vi "Main Low Level.vi"() -> ()   [LabVIEW 2015]
uses:
  <vilib>/userdefined/High Color/IMAQdx.ctl
  <vilib>/myRIO/Instrument Drivers/Onboard IO/UART/typedef/VISA Configuration.ctl
  <vilib>/Instr/_visa.llb/VISA Configure Serial Port (Instr).vi
  <vilib>/myRIO/Instrument Drivers/Onboard IO/UART/UART.lvlib
  <vilib>/vision/driver/NI_Vision_Acquisition_Software.lvlib
panel:
  out "NEW A":i32
  out "STOP STATE":dbl
  out "FRONT STATE":dbl
  out "LEFT STATE":dbl
  out "RIGHT STATE":dbl
  out "Buffer Number Out":u32
  in  "Session In":T1
  out "break stat":u16
  out "right stat":u16
  out "down stat":u16
  out "left stat":u16
  out "up stat":u16
  in  "stop":bool
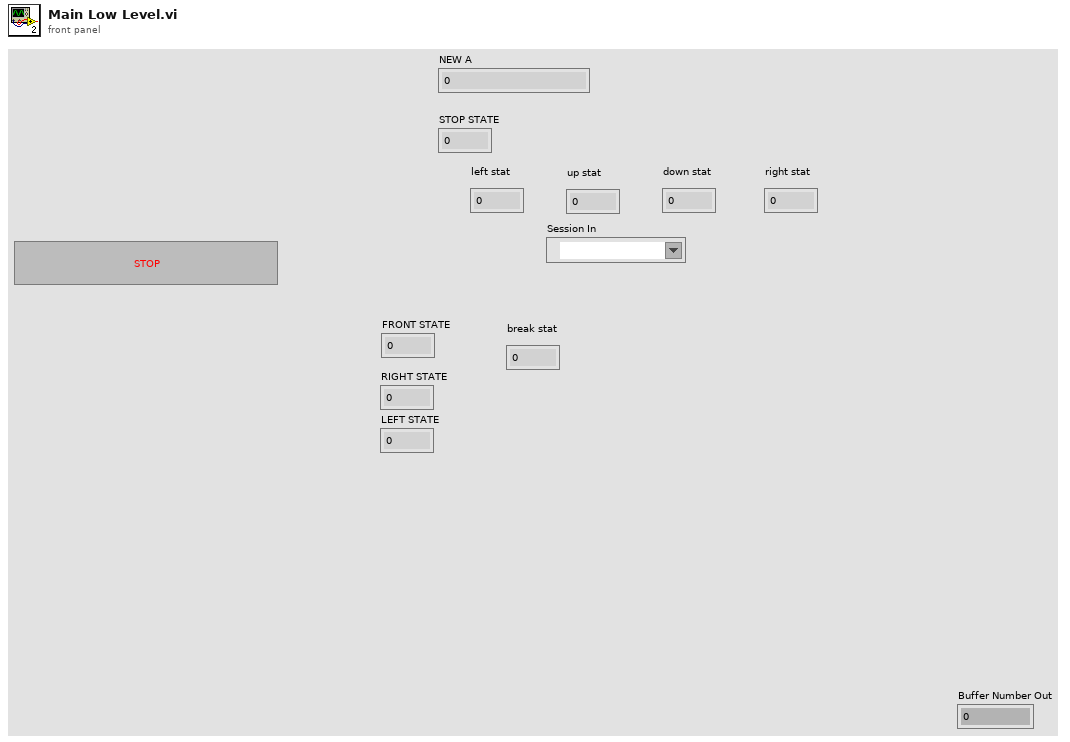
[diagram p1: front panel]
types:
  T1 = typedef "IMAQdx.ctl" = refnum<k21>
  T2 = typedef "Image Type" = u32
  T3 = typedef "UART.lvlib/VISA Configuration.ctl" = cluster{"baud rate (9600)":u32, "data bits (8)":u16, "parity (0:none)":enum16{"None", "Odd", "Even", "Mark", "Space"}, "stop bits (10: 1 bit)":u16, "flow control (0:none)":u16, "termination char\n(0xA = '\\n' = LF) ":u8, "Enable Termination\nChar (T)":bool, "timeout (10sec)":u32}
  T4 = typedef "IMAQ Image.ctl" = refnum<image>
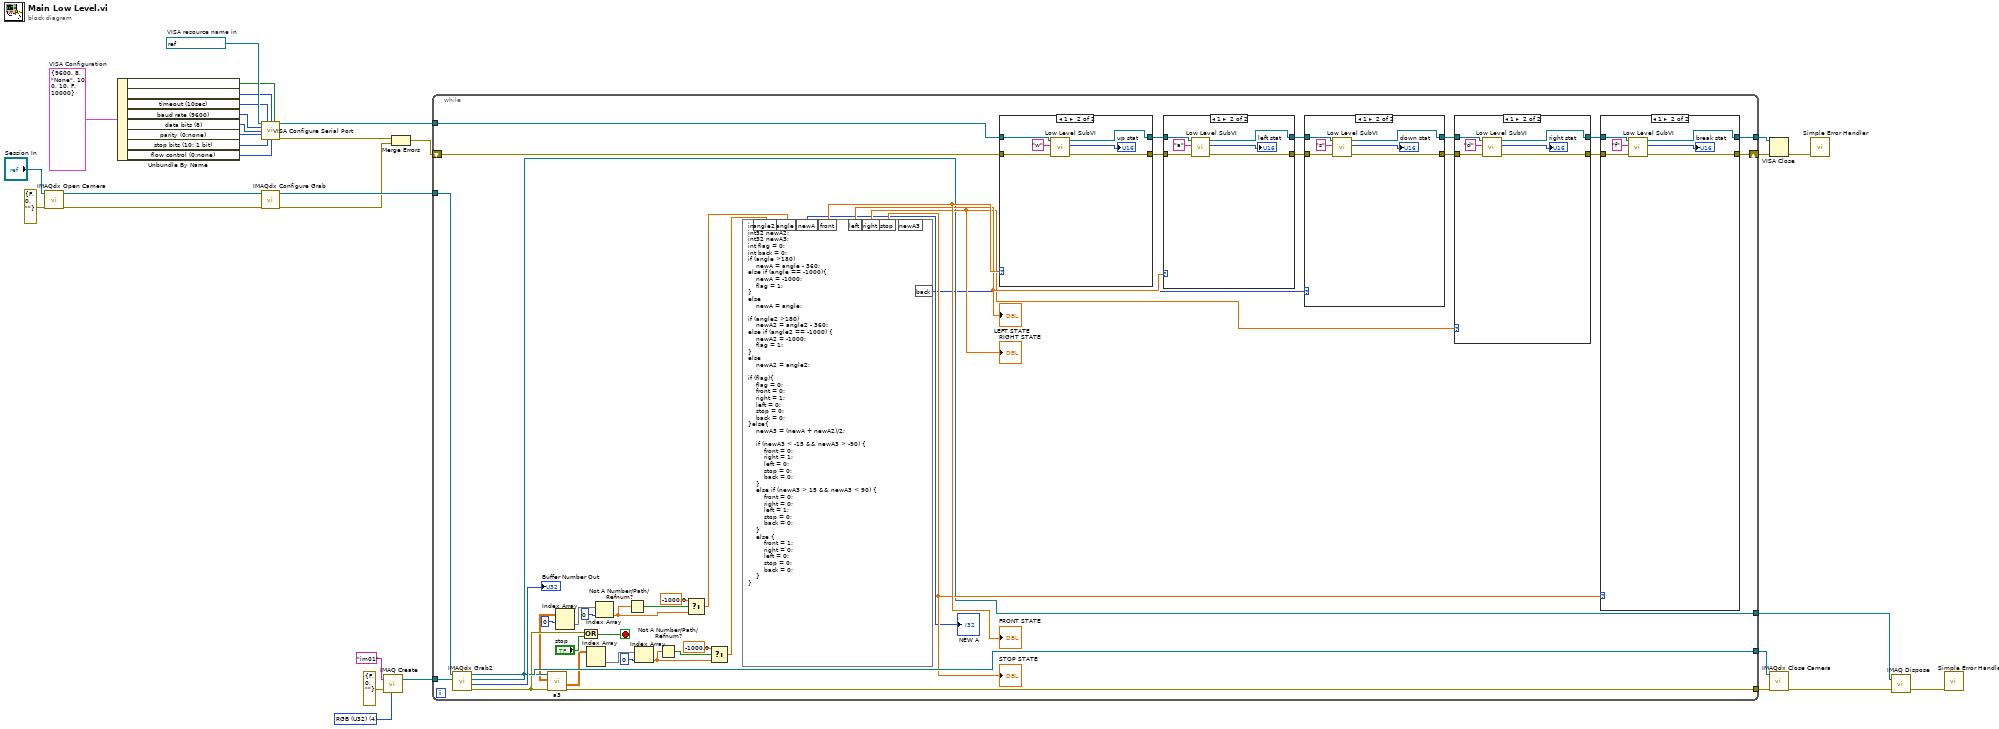
[diagram p0: block diagram]
diagram:
  w13 = T2 4 items=["Grayscale (U8)", "Grayscale (I16)", "Grayscale (SGL)", "Complex (CSG)", "RGB (U32)", "HSL (U32)", "RGB (U64)", "Grayscale (U16)"] ("Image Type")
  w30 = T3 {"baud rate (9600)"=9600, "data bits (8)"=8, "parity (0:none)"=enum."None", "stop bits (10: 1 bit)"=10, "flow control (0:none)"=0, "termination char\n(0xA = '\\n' = LF) "=10, "Enable Termination\nChar (T)"=FALSE, "timeout (10sec)"=10000}  # VISA Configuration
  w31 = refnum<visa-resource-name> "ASRL1::INSTR"  # VISA resource name in
  n1 = call <vilib>:"IMAQdx Open Camera.vi"("error in"=errorcluster {"status"=FALSE, "code"=0, "source"=""}, "Session In"="Session In") -> ("error out"=w16:errorcluster, "Session Out"=w17:T1)  [unwired: 8 in]
  n2 = Unbundle By Name(w30) -> ("Enable Termination\nChar (T)"=w29:bool, "termination char\n(0xA = '\\n' = LF)"=w28:u8, "timeout (10sec)"=w27:u32, "baud rate (9600)"=w22:u32, "data bits (8)"=w23:u16, "parity (0:none)"=w24:enum16{"None", "Odd", "Even", "Mark", "Space"}, "stop bits (10: 1 bit)"=w25:u16, "flow control (0:none)"=w26:u16)
  n3 = call-poly "VISA Configure Serial Port"("VISA resource name"=w31, "timeout (10sec)"=w27, "termination char\n(0xA = '\\n' = LF)"=w28, "Enable Termination\nChar (T)"=w29, "baud rate (9600)"=w22, "data bits (8)"=w23, "parity (0:none)"=w24, "stop bits (10: 1 bit)"=w25, "flow control (0:none)"=w26) -> ("VISA resource name out"=w21:refnum<visa-resource-name>, "error out"=w6:errorcluster)  [unwired: 5 in]
  n4 = call <vilib>:"IMAQdx Configure Grab.vi"("error in"=w16, "Session In"=w17) -> ("error out"=w7:errorcluster, "Session Out"=w8:T1)  [unwired: 8 in]
  n5 = call "IMAQ Create"("Image Name"="im01", "Image Type"=w13, "error in (no error)"=errorcluster {"status"=FALSE, "code"=0, "source"=""}) -> ("New Image"=w4:T4)  [unwired: 2 in, 1 out]
  n6 = Merge Errors(w6, w7) -> (w5:errorcluster)
  n7 = while {
    tunnel: w21 -> [w73]
    shift-right: [w57] -> w20
    shift-left: w5 -> [w72]
    tunnel: [w63] -> w19
    tunnel: w8 -> [w61]
    tunnel: w4 -> [w60]
    tunnel: [w44] -> w3
    tunnel: [w56] -> w2
    tunnel: [w43] -> w1
    stop <- w58 stop-if-true
    n8 = call <vilib>:"IMAQdx Grab2.vi"("Image In"=w60, "Session In"=w61) -> ("error out"=w45:errorcluster, "Buffer Number Out"=→"Buffer Number Out":u32, "Image Out"=w44:T4, "Session Out"=w56:T1)  [unwired: 6 in]
    n9 = call "a3.vi"("error in"=w45, "Image In"=w44) -> ("error out"=w43:errorcluster, "Calibrated Results (Caliper 2)"=w42:sgl[][], "Calibrated Results (Caliper 1)"=w41:sgl[][])  [unwired: 3 out]
    n10 = Index Array(array=w41, index (row)=0) -> (element=w51:sgl[])  [unwired: 1 in]
    n11 = Or(x=w45, y="stop") -> (x .or. y?=w58:bool)
    n12 = Index Array(array=w42) -> (element=w48:sgl[])  [unwired: 2 in]
    n13 = Index Array(array=w51, index=0) -> (element=w35:sgl)
    n14 = Not A Number/Path/Refnum?(number/path/refnum=w35) -> (NaN/Path/Refnum?=w36:bool)
    n15 = Index Array(array=w48, index=0) -> (element=w38:sgl)
    n16 = Not A Number/Path/Refnum?(number/path/refnum=w38) -> (NaN/Path/Refnum?=w39:bool)
    n17 = Select(t=-1000.0, s=w36, f=w35) -> (s? t:f=w34:dbl)
    n18 = Select(t=-1000.0, s=w39, f=w38) -> (s? t:f=w33:dbl)
    n19 = formula code="int32 newA;\nint32 newA2;\nint32 newA3;\nint flag = 0;\nint back = 0;\nif (angle >180)\n    newA = angle - 360;\nelse if (angle == -1000){\n    newA = -1000;\n    flag = 1;\n}\nelse\n    newA = angle;\n\nif (angle2 >180)\n    newA2 = angle2 - 360;\nelse if (angle2 == -1000) {\n    newA2 = -1000;\n    flag = 1;\n}\nelse\n    newA2 = angle2;\n\nif (flag){\n    flag = 0;\n    front = 0;\n    right = 1;\n    left = 0;\n    stop = 0;\n    back = 0;\n}else{\n    newA3 = (newA + newA2)/2;\n\n    if (newA3 < -15 && newA3 > -90) {\n        front = 0;\n        right = 1;\n        left = 0;\n        stop = 0;\n        back = 0;\n    }\n    else if (newA3 > 15 && newA3 < 90) {\n        front = 0;\n        right = 0;\n        left = 1;\n        stop = 0;\n        back = 0;\n    }\n    else {\n        front = 1;\n        right = 0;\n        left = 0;\n        stop = 0;\n        back = 0;\n    }\n}"("angle"=w34, "angle2"=w33) -> ("front"=w55:dbl, "left"=w54:dbl, "right"=w53:dbl, "stop"=w49:dbl, "newA"=→"NEW A":i32, "back"=w32:i32)  [unwired: 1 out]
    "RIGHT STATE" <- w53
    "LEFT STATE" <- w54
    "FRONT STATE" <- w55
    "STOP STATE" <- w49
    n20 = case shown="1" w55 {
      tunnel: w73 -> [w107 w111]
      tunnel: w72 -> [w106 w110]
      tunnel: [w107 w109] -> w71
      tunnel: [w106 w108] -> w70
      frame 0, Default {
      }
      frame 1 {
        n21 = call "Low Level SubVI.vi"("error in (no error)"=w110, "write buffer"="w", "VISA Refnum in"=w111) -> ("error out"=w108:errorcluster, "output 1"=→"up stat":u16, "VISA Refnum out"=w109:refnum<visa-resource-name>)  [unwired: 6 in]
      }
    }
    n22 = case shown="1" w54 {
      tunnel: w71 -> [w99 w103]
      tunnel: w70 -> [w98 w102]
      tunnel: [w99 w101] -> w69
      tunnel: [w98 w100] -> w68
      frame 0, Default {
      }
      frame 1 {
        n23 = call "Low Level SubVI.vi"("error in (no error)"=w102, "write buffer"="a", "VISA Refnum in"=w103) -> ("error out"=w100:errorcluster, "output 1"=→"left stat":u16, "VISA Refnum out"=w101:refnum<visa-resource-name>)  [unwired: 6 in]
      }
    }
    n24 = case shown="1" w32 {
      tunnel: w69 -> [w91 w92]
      tunnel: w68 -> [w90 w93]
      tunnel: [w91 w95] -> w67
      tunnel: [w90 w94] -> w66
      frame 0, Default {
      }
      frame 1 {
        n25 = call "Low Level SubVI.vi"("error in (no error)"=w93, "write buffer"="s", "VISA Refnum in"=w92) -> ("error out"=w94:errorcluster, "output 1"=→"down stat":u16, "VISA Refnum out"=w95:refnum<visa-resource-name>)  [unwired: 6 in]
      }
    }
    n26 = case shown="1" w53 {
      tunnel: w67 -> [w83 w84]
      tunnel: w66 -> [w82 w85]
      tunnel: [w83 w87] -> w65
      tunnel: [w82 w86] -> w64
      frame 0, Default {
      }
      frame 1 {
        n27 = call "Low Level SubVI.vi"("error in (no error)"=w85, "write buffer"="d", "VISA Refnum in"=w84) -> ("error out"=w86:errorcluster, "output 1"=→"right stat":u16, "VISA Refnum out"=w87:refnum<visa-resource-name>)  [unwired: 6 in]
      }
    }
    n28 = case shown="1" w49 {
      tunnel: w65 -> [w75 w77]
      tunnel: w64 -> [w74 w78]
      tunnel: [w75 w76] -> w63
      tunnel: [w74 w79] -> w57
      frame 0, Default {
      }
      frame 1 {
        n29 = call "Low Level SubVI.vi"("error in (no error)"=w78, "write buffer"="f", "VISA Refnum in"=w77) -> ("error out"=w79:errorcluster, "output 1"=→"break stat":u16, "VISA Refnum out"=w76:refnum<visa-resource-name>)  [unwired: 6 in]
      }
    }
  }
  n30 = VISA Close(VISA resource name=w19, error in (no error)=w20) -> (error out=w18:errorcluster)
  n31 = call <vilib>:"IMAQdx Close Camera.vi"("error in"=w1, "Session In"=w2) -> ("error out"=w10:errorcluster)  [unwired: 9 in]
  n32 = call <vilib>:"Simple Error Handler.vi"("error in (no error)"=w18) -> ()  [unwired: 4 in, 5 out]
  n33 = call "IMAQ Dispose"("Image"=w3, "error in (no error)"=w10) -> ("error out"=w9:errorcluster)  [unwired: 4 in]
  n34 = call <vilib>:"Simple Error Handler.vi"("error in (no error)"=w9) -> ()  [unwired: 4 in, 5 out]
